vi "PH_USB600x_AnalogReader.destructor.vi"(0 "i ref in":refnum<vi>, 5 "error in(no error)":errorcluster) -> (19 "error out":errorcluster)   [LabVIEW 2014, in "PH_USB600x_AnalogReader.lvlib"]
doc: "This is the destructor of a class.\n\nLicense Agreement for this software:\n\nCopyright (C)\nGesellschaft für Schwerionenforschung, GSI\nPlanckstr. 1\n64291 Darmstadt\nGermany\n\nContact: D.Beck@gsi.de \n\nThis program is free software; you can redistribute it and/or modify it under the terms of the \nGNU General Public License as published by the Free Software Foundation; either version 2 of \nthe license, or (at your option) any later version.\n\nThis program is distributed in the hope that it will be useful, but WITHOUT ANY WARRANTY; \nwithout even the implied warranty of MERCHANTABILITY or FITNESS FOR A PARTICULAR PURPOSE. See the GNU General License for more details (http://www.gnu.org).\n\nGesellschaft für Schwerionenforschung, GSI\nPlanckstr. 1, 64291 Darmstadt, Germany\nFor all questions and ideas contact: M.Richter@gsi.de, H.Brand@gsi.de or D.Beck@gsi.de.\nLast update: 16-JUN-2004"
uses:
  PH_USB600x_AnalogReader.lvlib
  CSApplicationBaseClasses/DeviceBase/DeviceBase.lvlib
  CSCore/BaseGUI/BaseGUI.lvlib
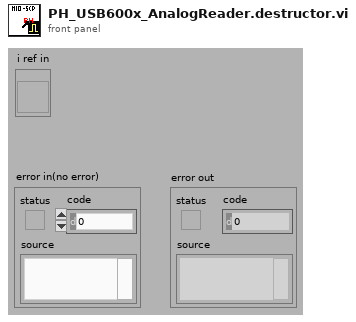
[diagram p1: front panel]
types:
  T1 = typedef "PH_USB600x_AnalogReader.lvlib/PH_USB600x_AnalogReader.i attribute.ctl" = cluster{"GUI Refs":cluster{"Delete":refnum<vi>, "Status":refnum<vi>, "Timeout":refnum<vi>, "Acquire Waveform":refnum<vi>, "Timing":refnum<vi>, "Graph":refnum<vi>, "Prdc Interval":refnum<vi>, "Formula":refnum<vi>}, "Device Settings":cluster{"AIChannel":refnum<k21>, "channelName":string, "Status":T2}, "Timing":T3, "Prdc Interval":dbl, "Lin Scaling":T4, "Data":cluster{"t0":timestamp, dbl}[]}
  T2 = typedef "PH_StatusHandler.lvlib/PH_StatusHandler.Status.ctl" = i16
  T3 = typedef "PH_USB600x_AnalogReader.lvlib/PH_USB600x_AnalogReader.Timing.ctl" = cluster{"Samples per Channel":i32, "Rate":dbl}
  T4 = typedef "PH_USB600x_AnalogReader.lvlib/PH_USB600x_AnalogReader.Lin Scaling.ctl" = cluster{"Slope [Unit/V]":dbl, "Offset [Unit]":dbl, "Y-Unit":string, "Y-Label":string}
  T5 = enum16{"SetAttribute", "GetAttribute", "CreateAttribute", "DestroyAttribute", "DestroyAllAtributes"}
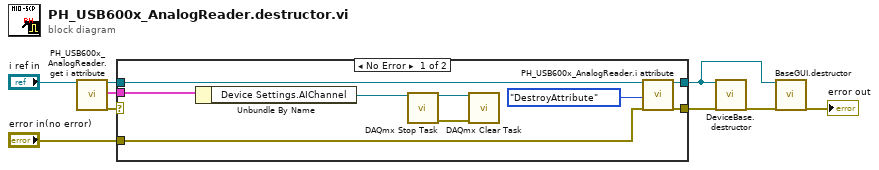
[diagram p0: block diagram]
diagram:
  n1 = call "PH_USB600x_AnalogReader.get i attribute.vi"("i ref in"="i ref in") -> ("i ref out"=w7:refnum<vi>, "i attribute"=w6:T1, "error out"=w5:errorcluster)  [unwired: 16 in]
  n2 = case shown="No Error" w5 {
    tunnel: [w17 w20] -> w1
    tunnel: [w16 w19] -> w9
    tunnel: w7 -> [w15 w20]
    tunnel: w6 -> [w14 _]
    tunnel: "error in(no error)" -> [w10 w19]
    frame No Error {
      n3 = Unbundle By Name(w14) -> ("Device Settings.AIChannel"=w11:refnum<k21>)
      n4 = call <vilib>:"DAQmx Stop Task.vi"("task/channels in"=w11) -> ("task out"=w13:refnum<k21>, "error out"=w12:errorcluster)  [unwired: 13 in]
      n5 = call <vilib>:"DAQmx Clear Task.vi"("task in"=w13, "error in"=w12) -> ()  [unwired: 13 in, 1 out]
      n6 = call "PH_USB600x_AnalogReader.i attribute.vi"("VI Refnum"=w15, "Action"=T5."DestroyAttribute", "error in (no error)"=w10) -> ("VI Refnum out"=w17:refnum<vi>, "error out"=w16:errorcluster)  [unwired: 14 in, 1 out]
    }
    frame Error {
    }
  }
  n7 = call "DeviceBase.destructor.vi"("i ref in"=w1, "error in (no error)"=w9) -> ("error out"=w3:errorcluster)  [unwired: 17 in]
  n8 = call "BaseGUI.destructor.vi"("i ref in"=w1, "error in (no error)"=w3) -> ("error out"=→"error out":errorcluster)  [unwired: 17 in]
